vi "Cycle Duration Edit steptypes.vi"(8 "error in":errorcluster, 10 "Cycle Duration Data in":T1, 11 "Sequence Context In":refnum<k7>) -> (0 "error out":errorcluster, 2 "Cycle Duration Data out":T1)   [LabVIEW 2023, in "LTT_TeststandSteptypes.lvlib"]
uses:
  LTT_TeststandSteptypes.lvlib
  Control/Cycle Duration Selection.ctl
  Control/Cycle Duration Data.ctl
  <vilib>/addons/TestStand/_TSUtility.llb/TestStand - Start Modal Dialog (Sequence Context).vi
  <vilib>/addons/TestStand/_TSUtility.llb/TestStand - End Modal Dialog (Sequence Context).vi
  HardwareAbstractionLayer_LVOOP/Database/Database.lvclass
  HardwareAbstractionLayer_LVOOP/Database/SQL Public VI/Control/DB Options.ctl
panel:
  in  "CYCLE_DURATION_LOG":T2
  in  "Close":bool
  in  "OK":bool
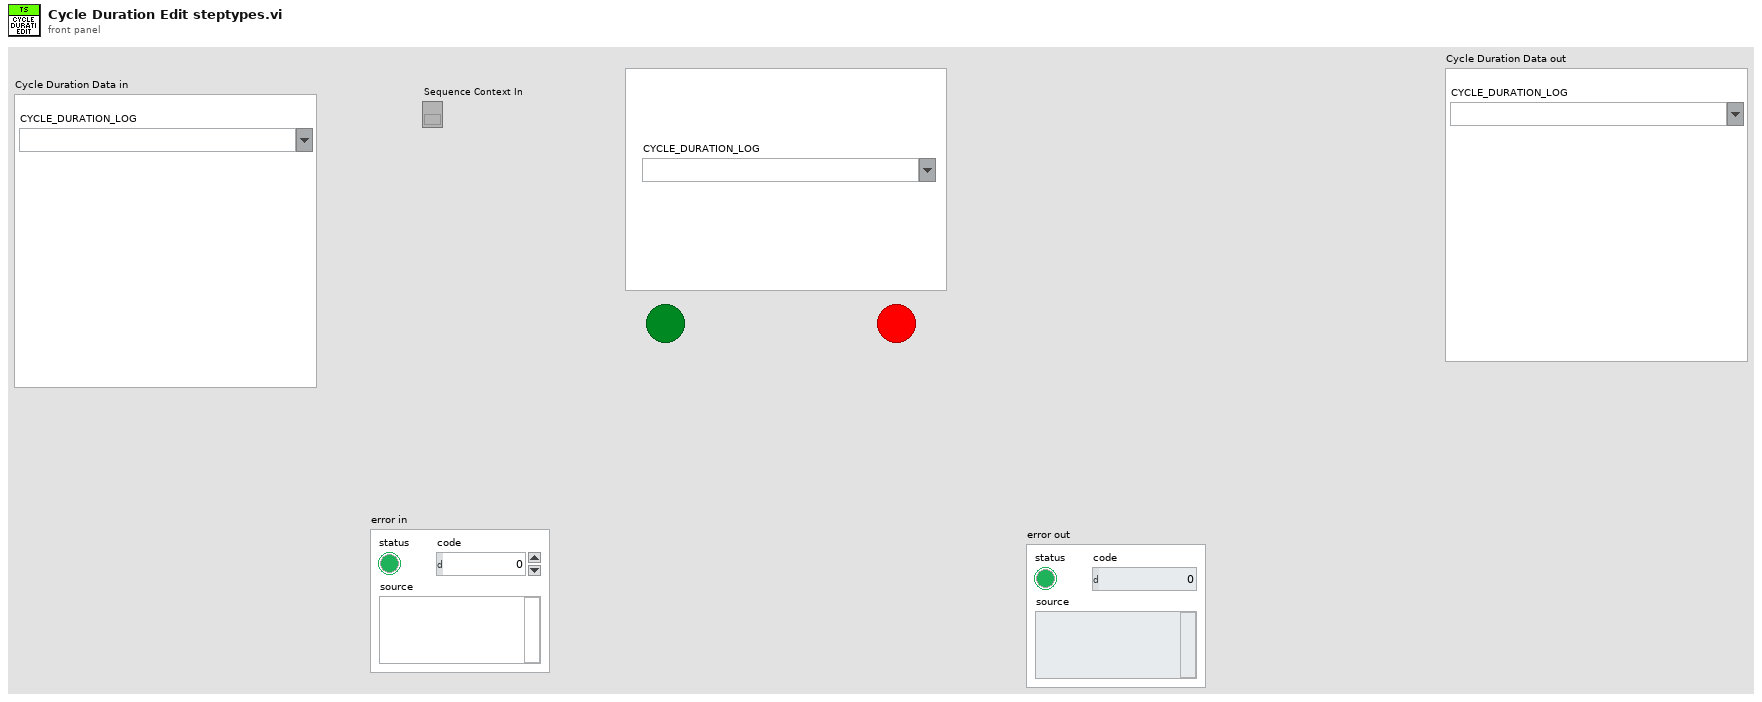
[diagram p1: front panel]
types:
  T1 = typedef "LTT_TeststandSteptypes.lvlib/Cycle Duration Data.ctl" = cluster{"CYCLE_DURATION_LOG":T2}
  T2 = typedef "LTT_TeststandSteptypes.lvlib/Cycle Duration Selection.ctl" = string
  T3 = typedef "HardwareAbstractionLayer_LVOOP.lvlib/Database.lvclass/DB Options.ctl" = enum16{"Init", "Select Data", "Insert Data", "Update Data", "Delete Data", "Execute Query", "Create Schema", "Create Table", "List Tables", "List Columns", "Close"}
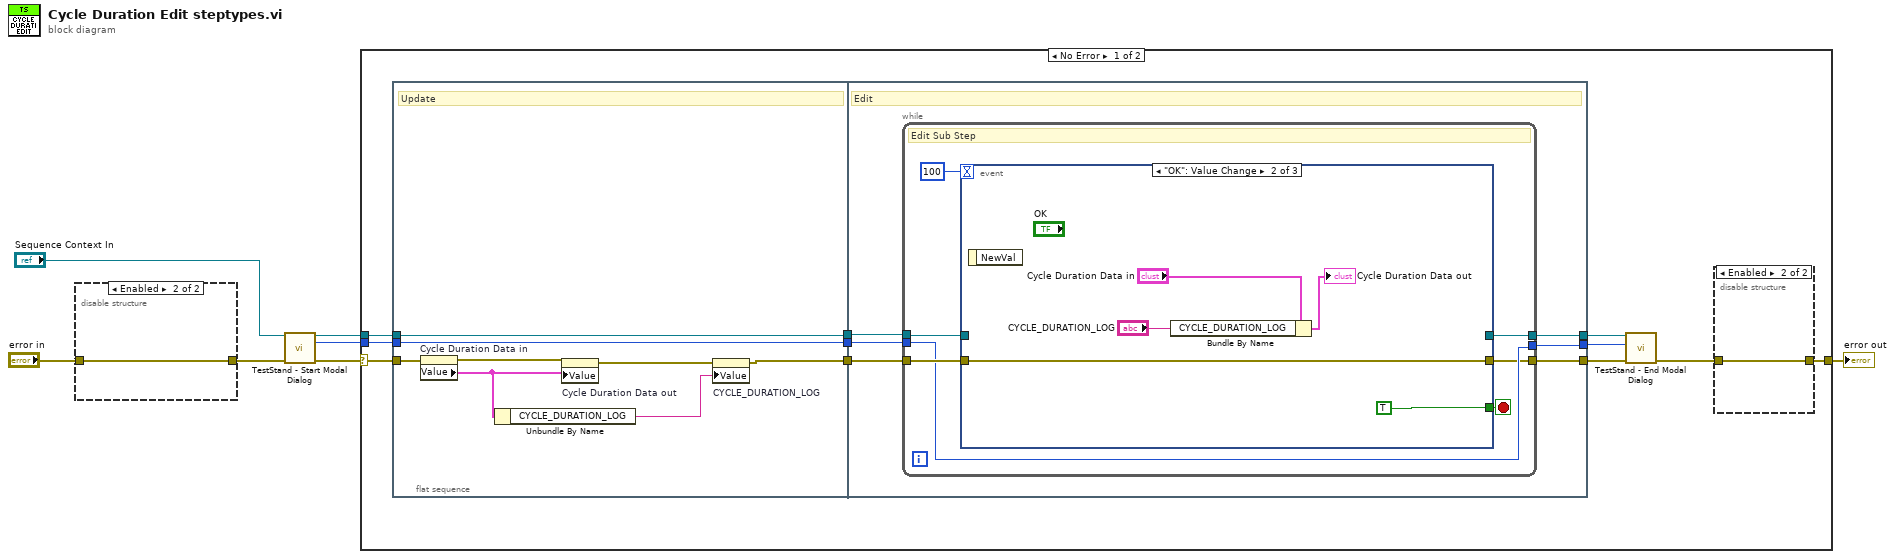
[diagram p0: block diagram]
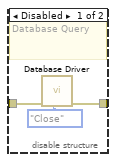
[diagram p2: hidden frame]
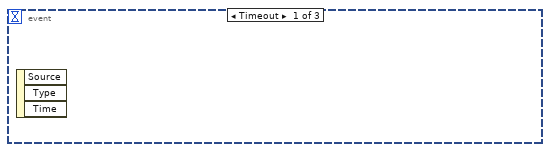
[diagram p3: hidden frame]
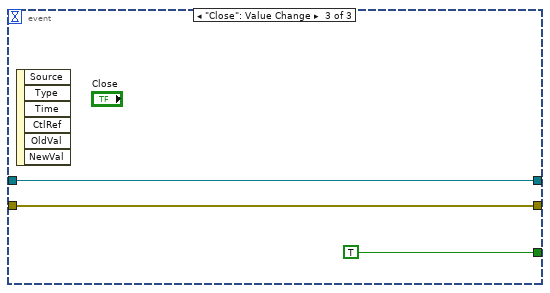
[diagram p4: hidden frame]
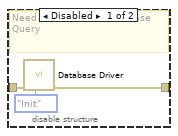
[diagram p6: hidden frame]
diagram:
  n1 = disable-structure shown="Enabled" {
    disable-tunnel: "error in" -> [w10 w11]
    disable-tunnel: [w9 w11] -> w2
    frame Disabled {
      # "Need to Enable for Database Query"
      n2 = call "Database Driver.vi"("Options"=DB_Options."Init", "error in"=w10) -> ("error out"=w9:errorcluster)  [unwired: 6 in, 3 out]
    }
    frame Enabled {
    }
  }
  n3 = call-poly <vilib>:"TestStand - Start Modal Dialog.vi"("Sequence Context In"="Sequence Context In", "error in (no error)"=w2) -> ("Sequence Context Out"=w4:refnum<k7>, "Modal ID"=w3:i32, "error out"=w5:errorcluster)  [unwired: 9 in, 2 out]
  n4 = case shown="No Error" w5 {
    selector: w5 -> [w19 w56]
    tunnel: w4 -> [w16 _]
    tunnel: w3 -> [w15 _]
    tunnel: [w12 w56] -> w1
    frame No Error {
      n5 = flat-sequence {
        tunnel: w19 -> [w32]
        tunnel: [w28] -> w22
        tunnel: w16 -> [w34]
        tunnel: w15 -> [w33]
        tunnel: [w34] -> w21
        tunnel: [w33] -> w20
        tunnel: w22 -> [w38]
        tunnel: [w36] -> w18
        tunnel: w21 -> [w40]
        tunnel: w20 -> [w39]
        tunnel: [w37] -> w14
        tunnel: [w35] -> w13
        frame #0 {
          # "Update"
          n6 = property on="Cycle Duration Data in" class="Clust (strict)"(error in=w32) -> (error out=w31:errorcluster, "Value"=w30:T1)  [unwired: 1 in, 1 out]
          n7 = Unbundle By Name(w30) -> ("CYCLE_DURATION_LOG"=w27:T2)
          n8 = property on="Cycle Duration Data out" class="Clust (strict)"(error in=w31, "Value"=w30) -> (error out=w29:errorcluster)  [unwired: 1 in, 1 out]
          n9 = property on="CYCLE_DURATION_LOG" class="CmbBox (strict)"(error in=w29, "Value"=w27) -> (error out=w28:errorcluster)  [unwired: 1 in, 1 out]
        }
        frame #1 {
          # "Edit"
          n10 = while {
            tunnel: w40 -> [w45]
            tunnel: w39 -> [w42]
            tunnel: w38 -> [w43]
            tunnel: [w44] -> w35
            tunnel: [w42] -> w37
            tunnel: [w41] -> w36
            stop <- w46 stop-if-true
            # "Edit Sub Step"
            n11 = event shown="[1] \"OK\": Value Change" {
              selector: _ -> [_ _ _]
              dyn-events: _ -> [_ _ _]
              timeout: 100 -> [_ _ _]
              tunnel: [_ TRUE TRUE] -> w46
              tunnel: [_ _ w54] -> w44
              tunnel: w45 -> [_ _ w54]
              tunnel: w43 -> [_ w51 w53]
              tunnel: [_ w51 w53] -> w41
              event Timeout {
                n12 = event-data() -> ()  [unwired: 1 in, 3 out]
              }
              event "OK": Value Change {
                n13 = event-data() -> ()  [unwired: 1 in, 1 out]
                n14 = Bundle By Name(cluster="Cycle Duration Data in", "CYCLE_DURATION_LOG"="CYCLE_DURATION_LOG") -> (→"Cycle Duration Data out":T1)
              }
              event "Close": Value Change {
                n15 = event-data() -> ()  [unwired: 1 in, 6 out]
              }
            }
          }
        }
      }
      n16 = call-poly <vilib>:"TestStand - End Modal Dialog.vi"("Sequence Context In"=w13, "Modal ID"=w14, "error in (no error)"=w18) -> ("error out"=w17:errorcluster)  [unwired: 12 in]
      n17 = disable-structure shown="Enabled" {
        disable-tunnel: w17 -> [w25 w26]
        disable-tunnel: [w24 w26] -> w12
        frame Disabled {
          # "Need to Enable for Database Query"
          n18 = call "Database Driver.vi"("Options"=DB_Options."Close", "error in"=w25) -> ("error out"=w24:errorcluster)  [unwired: 6 in, 3 out]
        }
        frame Enabled {
        }
      }
    }
    frame Error {
    }
  }
  "error out" <- w1
